vi "Pkt - Packet Type.vi"(6 "Buffered?":bool, 8 "error in (no error)":errorcluster, 11 "Item Ref in":T2 format="%.0x") -> (0 "error out":errorcluster, 2 "Packet Type":T1, 3 "Item Ref out":T2 format="%.0x")   [LabVIEW 2016, in "UDP-Custom-Device System Explorer.lvlib"]
uses:
  UDP-Custom-Device System Explorer.lvlib
  <vilib>/NI Veristand/Custom Device API/Custom Device Item Ref.ctl
  Types/Packet Info/Packet Type.ctl
  <vilib>/NI VeriStand/Custom Device API/Custom Device API.lvlib
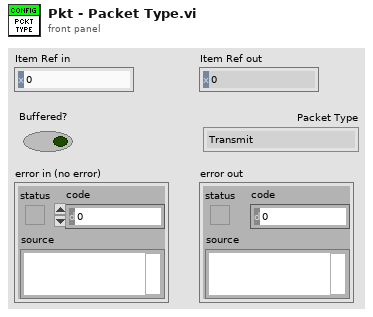
[diagram p1: front panel]
types:
  T1 = typedef "UDP-Custom-Device System Explorer.lvlib/Packet Type.ctl" = enum16{"Transmit", "Receive", "Buffered Transmit", "Buffered Receive"}
  T2 = typedef "Custom Device API.lvlib/Custom Device Item Ref.ctl" = u64
  T3 = typedef "Custom Device API.lvlib/Custom Device Item Info.ctl" = cluster{"Name":string, "Is Channel":bool, "GUID":string, "Is Waveform":bool}
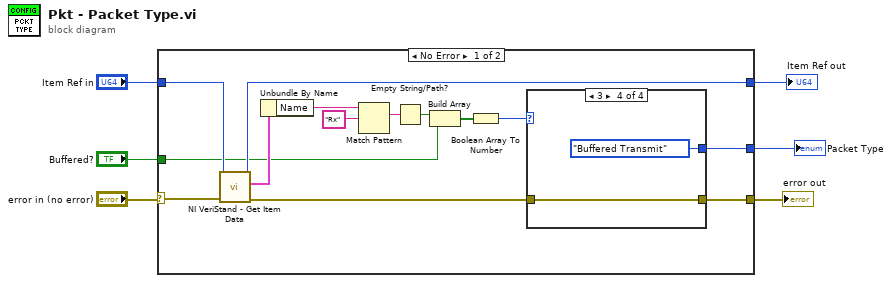
[diagram p0: block diagram]
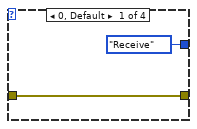
[diagram p2: hidden frame]
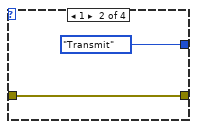
[diagram p3: hidden frame]
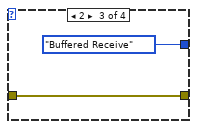
[diagram p4: hidden frame]
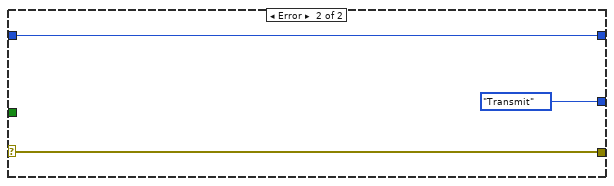
[diagram p5: hidden frame]
diagram:
  n1 = case shown="No Error" "error in (no error)" {
    selector: "error in (no error)" -> [w18 w31]
    tunnel: [w10 w31] -> w6
    tunnel: "Item Ref in" -> [w16 w30]
    tunnel: [w15 w30] -> w3
    tunnel: "Buffered?" -> [w13 _]
    tunnel: [w8 Packet_Type."Transmit" ("Packet Type")] -> w1
    frame No Error {
      n2 = call <vilib>:"NI VeriStand - Get Item Data.vi"("error in (no error)"=w18, "Item Ref in"=w16) -> ("error out"=w9:errorcluster, "Item Info"=w19:T3, "Item Ref out"=w15:T2)  [unwired: 6 in, 1 out]
      n3 = Unbundle By Name(w19) -> ("Name"=w7:string)
      n4 = Match Pattern(string=w7, regular expression="Rx") -> (match substring=w17:string)  [unwired: 1 in, 3 out]
      n5 = Empty String/Path?(string/path=w17) -> (empty?=w14:bool)
      n6 = Build Array(w14, w13) -> (w12:bool[])
      n7 = Boolean Array To Number(Boolean array=w12) -> (number=w11:u32)
      n8 = case shown="3" w11 {
        tunnel: [w22 w23 w26 w28] -> w10
        tunnel: w9 -> [w22 w23 w26 w28]
        tunnel: [Packet_Type."Receive" ("Packet Type") Packet_Type."Transmit" ("Packet Type") Packet_Type."Buffered Receive" ("Packet Type") Packet_Type."Buffered Transmit" ("Packet Type")] -> w8
        frame 0, Default {
        }
        frame 1 {
        }
        frame 2 {
        }
        frame 3 {
        }
      }
    }
    frame Error {
    }
  }
  "error out" <- w6
  "Packet Type" <- w1
  "Item Ref out" <- w3
